vi "PH_PowerUnit_BaseClass.Switch PU on GUI element.vi"(0 "i ref in":refnum<vi>, 2 "PU on (off)":bool, 5 "error in (no error)":errorcluster) -> (14 "i ref out":refnum<vi>, 19 "error out":errorcluster)   [LabVIEW 2014]
doc: "This VI sets the PU on GUI element."
uses:
  PH_PowerUnit_BaseClass.lvlib
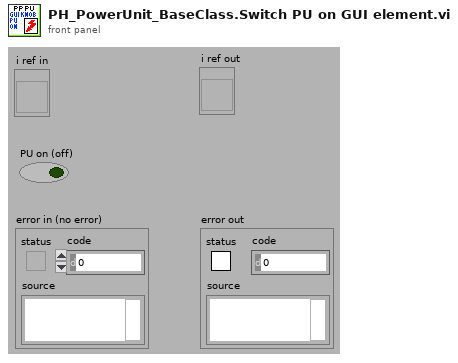
[diagram p1: front panel]
types:
  T1 = typedef "PH_PowerUnit_BaseClass.lvlib/PH_PowerUnit_BaseClass.i attribute.ctl" = cluster{"Constructor finished":bool, "PU":cluster{"In use":bool, "GUI Ref":refnum<vi>}, "Enabling":cluster{"State":T2, "GUI Ref":refnum<vi>}, "Subscribed Stati":cluster{"Instancename":string, "Status":T3, "linked?":bool, "Shot Condition":T3, "GUI Ref":refnum<vi>}[], "Timing":cluster{"Last Shot":dbl, "Time between Shots [Sec]":dbl, "Waiting Time over?":bool, "Service ID Waiting Time":i32, "GUI Ref":refnum<vi>}, "Sequencer":cluster{"Instance":string, "SM State":string, "GUI Ref":refnum<vi>}, "Status":cluster{"Status":T3, "Service ID":i32, "GUI Ref":refnum<vi>}}
  T2 = typedef "Enabling State.ctl" = i32
  T3 = typedef "Status.ctl" = i16
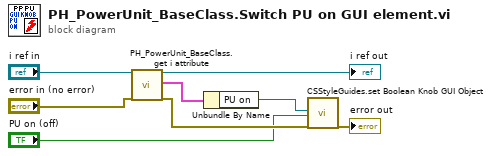
[diagram p0: block diagram]
diagram:
  n1 = call "PH_PowerUnit_BaseClass.get i attribute.vi"("i ref in"="i ref in", "error in (no error)"="error in (no error)") -> ("i ref out"=→"i ref out":refnum<vi>, "i attribute"=w6:T1, "error out"=w3:errorcluster)  [unwired: 15 in]
  n2 = Unbundle By Name(w6) -> ("PU on"=w4:refnum<vi>)
  n3 = call "CSStyleGuides.set Boolean Knob GUI Object.vi"("Boolean Knob GUI Ref"=w4, "Value"="PU on (off)", "error in (no error)"=w3) -> ("error out"=→"error out":errorcluster)  [unwired: 16 in]
